vi "departure.vi"() -> ()   [LabVIEW 2014]
panel:
  out "departure":string
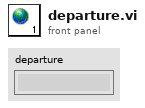
[diagram p1: front panel]
diagram:
